vi "Read Pipeline.vi"(8 "error in (no error)":errorcluster, 11 "Redis Pipelining Client in":refnum<class "Redis Pipelining TCP Client.lvclass">) -> (0 "error out":errorcluster, 1 "remaning values":i32, 2 "RESP3 Values":variant[](array[variant]), 3 "Redis Pipelining Client out":refnum<class "Redis Pipelining TCP Client.lvclass">)   [LabVIEW 2019, in "Redis Client for LabVIEW.lvlib" / "Redis Pipelining TCP Client.lvclass"]
uses:
  Redis Pipelining TCP Client.lvclass
  Redis Pipelining TCP Client.lvclass/Redis Pipelining TCP Client.ctl
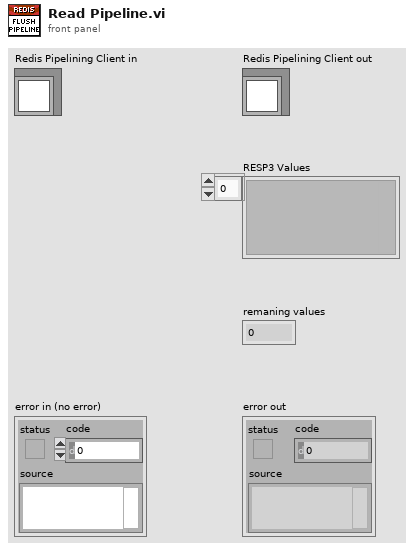
[diagram p1: front panel]
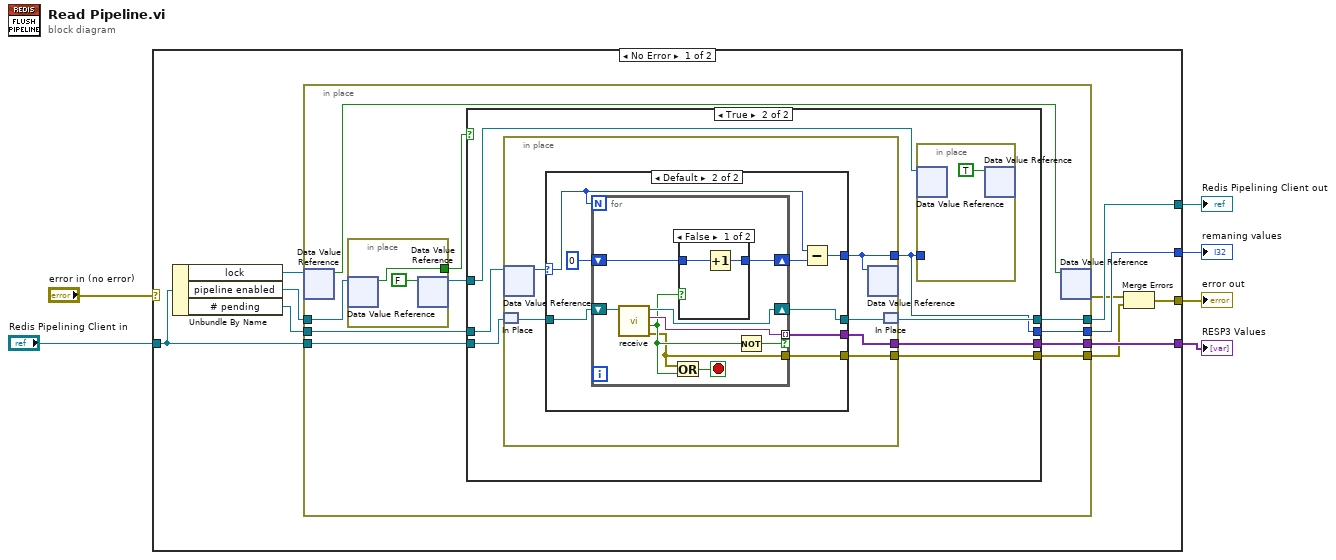
[diagram p0: block diagram]
diagram:
  n1 = case shown="No Error" "error in (no error)" {
    selector: "error in (no error)" -> [_ w67]
    tunnel: [w8 w67] -> w5
    tunnel: [w12 w66] -> w3
    tunnel: "Redis Pipelining Client in" -> [w15 w66]
    tunnel: [w14 _] -> w2
    tunnel: [w13 _] -> w1
    frame No Error {
      n2 = Unbundle By Name(w15) -> ("lock"=w10:refnum<data-value>, "pipeline enabled"=w11:refnum<data-value>, "# pending"=w16:refnum<data-value>)
      n3 = in-place {
        in-place-border: w16 -> [w26]
        in-place-border: w15 -> [w25]
        in-place-border: [w24] -> w14
        in-place-border: [w23] -> w13
        in-place-border: [w22] -> w12
        in-place-border: w11 -> [w21]
        in-place-border: [w17] -> w7
        n4 = in-place-dvr #1(w10) -> (w18:bool)  [unwired: 1 out]
        n5 = in-place {
          in-place-border: [w64] -> w20
          n6 = in-place-dvr #2(w21) -> (w64:bool)  [unwired: 1 out]
          n7 = in-place-dvr #2(FALSE) -> (w19:refnum<data-value>)  [unwired: 1 out]
        }
        n8 = case shown="True" w20 {
          tunnel: w26 -> [_ w34]
          tunnel: w25 -> [w27 w33]
          tunnel: [_ w29] -> w24
          tunnel: [_ w32] -> w23
          tunnel: [w27 w31] -> w22
          tunnel: w19 -> [_ w30]
          tunnel: [_ w28] -> w17
          frame False {
          }
          frame True {
            n9 = in-place {
              in-place-border: [w38] -> w29
              in-place-border: [w37] -> w32
              in-place-border: [w36] -> w28
              n10 = in-place-dvr #3(w34) -> (w41:i32)  [unwired: 1 out]
              n11 = in-place-match #4(w33) -> (w40:refnum<class "Redis Pipelining TCP Client.lvclass">)
              n12 = case shown="Default" w41 {
                selector: w41 -> [w42 w49]
                tunnel: w40 -> [w43 w51]
                tunnel: [w43 w50] -> w39
                tunnel: [w42 w47] -> w38
                tunnel: [_ w45] -> w37
                tunnel: [_ w44] -> w36
                frame 0 {
                }
                frame Default {
                  n13 = for {
                    N: w49 -> [_]
                    shift-right: [w59] -> w50
                    shift-left: w51 -> [w60]
                    tunnel: [w58] -> w45 mode=indexing if=w57
                    shift-right: [w55] -> w48
                    shift-left: 0 -> [w54]
                    tunnel: [w52] -> w44
                    stop <- w53 stop-if-true
                    n14 = call-dynamic "receive.vi"("Redis Pipelining TCP Client in"=w60) -> ("error out"=w52:errorcluster, "timed out?"=w56:bool, "RESP3 Value"=w58:variant, "Redis Pipelining TCP Client out"=w59:refnum<class "Redis Pipelining TCP Client.lvclass">)  [unwired: 7 in]
                    n15 = Or(x=w52, y=w56) -> (x .or. y?=w53:bool)
                    n16 = case shown="False" w56 {
                      tunnel: [w62 w63] -> w55
                      tunnel: w54 -> [w61 w63]
                      frame False {
                        n17 = Increment(x=w61) -> (x+1=w62:i32)
                      }
                      frame True {
                      }
                    }
                    n18 = Not(x=w56) -> (.not. x?=w57:bool)
                  }
                  n19 = Subtract(x=w49, y=w48) -> (x-y=w47:i32)
                }
              }
              n20 = in-place-dvr #3(w38) -> ()  [unwired: 2 out]
              n21 = in-place-match #4(w39) -> (w31:refnum<class "Redis Pipelining TCP Client.lvclass">)
            }
            n22 = in-place {
              in-place-border: w29 -> [_]
              n23 = in-place-dvr #5(w30) -> ()  [unwired: 2 out]
              n24 = in-place-dvr #5(TRUE) -> ()  [unwired: 2 out]
            }
          }
        }
        n25 = in-place-dvr #1(w18) -> (w9:errorcluster)  [unwired: 1 out]
      }
      n26 = Merge Errors(w9, w7) -> (w8:errorcluster)
    }
    frame Error {
    }
  }
  "error out" <- w5
  "Redis Pipelining Client out" <- w3
  "remaning values" <- w2
  "RESP3 Values" <- w1
